vi "1.2.1.3-Gen RW Receive Case.vi"(3 "Local Clock: Clk":i8, 4 "Foreign Clock: Clk*":i8, 5 "RS232-1\\Port1 Write Timeout":bool) -> (0 "New Local Clock: Clk":i8, 1 "State":T1(ring), 2 "RS232-1\\Port1 Write":bool)   [LabVIEW 2010]
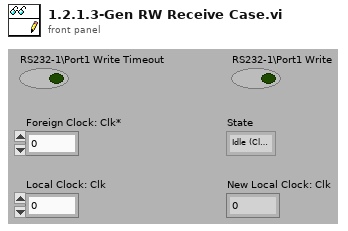
[diagram p1: front panel]
types:
  T1 = enum8{"Idle (Clk=-1)", "Sending(Clk*==Clk+1?Clk=Clk*:;)", "Receiving(Clk*==Clk?Clk++:;)"}
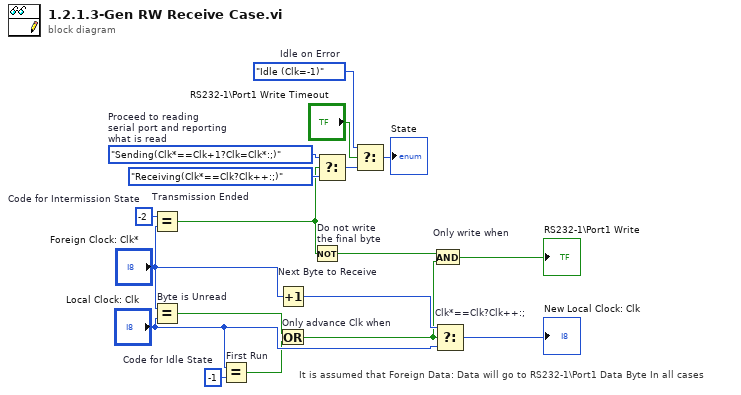
[diagram p0: block diagram]
diagram:
  w5 = i8 -2  # Code for Intermission State
  w16 = i8 -1  # Code for Idle State
  w14 = T1."Idle (Clk=-1)"  # Idle on Error
  w9 = T1."Sending(Clk*==Clk+1?Clk=Clk*:;)"  # Proceed to reading serial port and reporting what is read
  # "It is assumed that Foreign Data: Data will go to RS232-1\\Port1 Data Byte In all cases"
  n1 = Equal? "Transmission Ended"(x=w5, y="Foreign Clock: Clk*") -> (x = y?=w1:bool)
  n2 = Equal? "Byte is Unread"(x="Foreign Clock: Clk*", y="Local Clock: Clk") -> (x = y?=w12:bool)
  n3 = Equal? "First Run"(x="Local Clock: Clk", y=w16) -> (x = y?=w3:bool)
  n4 = Increment "Next Byte to Receive"(x="Foreign Clock: Clk*") -> (x+1=w10:i8)
  n5 = Or "Only advance Clk when"(x=w12, y=w3) -> (x .or. y?=w7:bool)
  n6 = Not "Do not write\nthe final byte"(x=w1) -> (.not. x?=w2:bool)
  n7 = Select(t=w9, s=w1, f=T1."Receiving(Clk*==Clk?Clk++:;)" ("State")) -> (s? t:f=w13:T1)
  n8 = Select(t=w14, s="RS232-1\\Port1 Write Timeout", f=w13) -> (s? t:f=→"State":T1)
  n9 = And "Only write when"(x=w2, y=w7) -> (x .and. y?=→"RS232-1\\Port1 Write":bool)
  n10 = Select "Clk*==Clk?Clk++:;"(t=w10, s=w7, f="Local Clock: Clk") -> (s? t:f=→"New Local Clock: Clk":i8)
